vi "ConfigActor.vi"(10 "Alias":string, 11 "Actor":refnum<class "Actor.lvclass">) -> (3 "ActorMap":T1)   [LabVIEW 2020, in "jettl.lvlib"]
uses:
  jettl.lvlib
  Actor/Actor.lvclass
  ActorMap.ctl
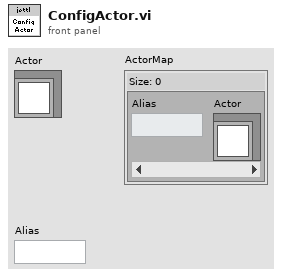
[diagram p1: front panel]
types:
  T1 = typedef "jettl.lvlib/ActorMap.ctl" = map{string, refnum<class "Actor.lvclass">}
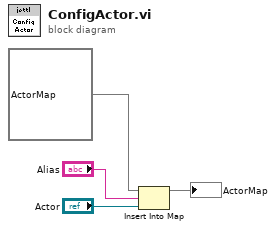
[diagram p0: block diagram]
diagram:
  n1 = Insert Into Map(map in=T1 {} ("ComponentActorAlias"), key="Alias", value="Actor") -> (map out=→"ActorMap":T1)  [unwired: 2 out]
